vi "MISC Get Path Information.vi"(11 "Error In (no error)":errorcluster) -> (3 "Top Level VI Name":string, 4 "Root Drive":path, 6 "Application Directory":path, 8 "Support Directory":path, 10 "Top Level VI Path":path, 14 "Development Environment":bool, 15 "Error Out":errorcluster)   [LabVIEW 2017]
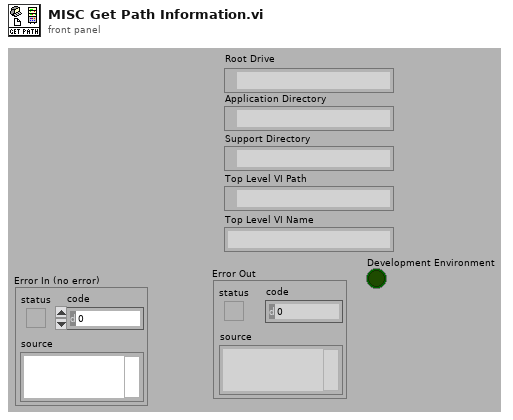
[diagram p1: front panel]
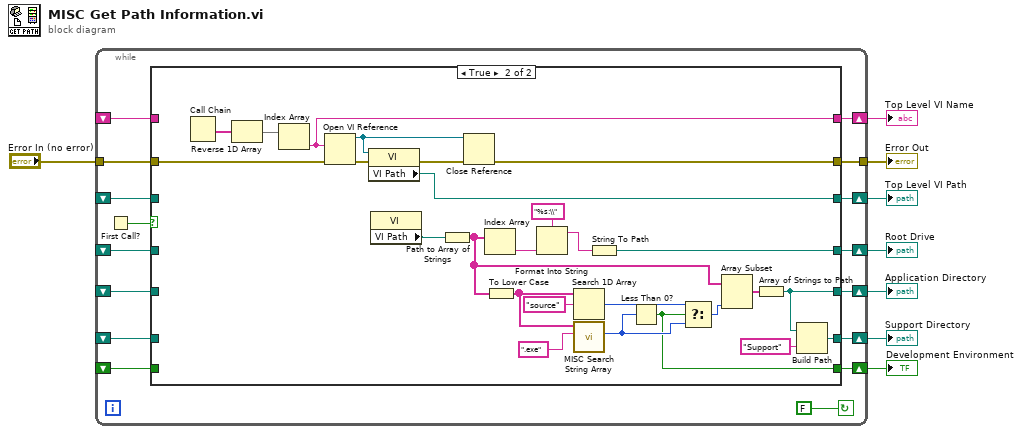
[diagram p0: block diagram]
diagram:
  n1 = while {
    tunnel: "Error In (no error)" -> [w24]
    tunnel: [w23] -> w7
    shift-right: [w17] -> w3
    shift-left: _ -> [w12]
    shift-right: [w18] -> w4
    shift-left: _ -> [w13]
    shift-right: [w19] -> w5
    shift-left: _ -> [w14]
    shift-right: [w20] -> w6
    shift-left: _ -> [w15]
    shift-right: [w21] -> w2
    shift-left: _ -> [w16]
    shift-right: [w10] -> w1
    shift-left: _ -> [w9]
    stop <- FALSE continue-if-true
    n2 = First Call?() -> (First Call?: T/F=w22:bool)
    n3 = case shown="True" w22 {
      tunnel: [w28 w57] -> w19
      tunnel: [w31 w54] -> w21
      tunnel: w24 -> [w29 w50]
      tunnel: [w29 w49] -> w23
      tunnel: [w27 w47] -> w18
      tunnel: [w26 w45] -> w17
      tunnel: [w30 w32] -> w20
      tunnel: w16 -> [w31 _]
      tunnel: w15 -> [w30 _]
      tunnel: w14 -> [w28 _]
      tunnel: w13 -> [w27 _]
      tunnel: w12 -> [w26 _]
      tunnel: [w25 w34] -> w10
      tunnel: w9 -> [w25 _]
      frame False {
      }
      frame True {
        n4 = Call Chain() -> (call chain=w56:string[])
        n5 = Reverse 1D Array(array=w56) -> (reversed array=w55:string[])
        n6 = Index Array(array=w55) -> (element=w54:string)  [unwired: 1 in]
        n7 = Open VI Reference(vi path=w54, error in (no error)=w50) -> (vi reference=w51:refnum<vi>, error out=w53:errorcluster)  [unwired: 4 out]
        n8 = property class="VI"(reference=w51, error in=w53) -> (error out=w52:errorcluster, "VI Path"=w32:path)  [unwired: 1 out]
        n9 = property class="VI"() -> ("VI Path"=w33:path)  [unwired: 2 in, 2 out]
        n10 = Path to Array of Strings(0:w33) -> (2:w44:string[])  [unwired: 1 out]
        n11 = Close Reference(reference=w51, error in (no error)=w52) -> (error out=w49:errorcluster)
        n12 = Index Array(array=w44) -> (element=w36:string)  [unwired: 1 in]
        n13 = To Lower Case(string=w44) -> (all lower case string=w42:string[])
        n14 = Format Into String(format string="%s:\\", w36) -> (resulting string=w35:string)  [unwired: 2 in, 1 out]
        n15 = Search 1D Array(1D array=w42, element="source") -> (index of element=w39:i32)  [unwired: 1 out]
        n16 = call "MISC Search String Array.vi"("String"=".exe" ("element"), "String Array"=w42) -> ("First Index"=w38:i32)  [unwired: 1 in, 8 out]
        n17 = String To Path(string=w35) -> (path=w57:path)
        n18 = Less Than 0?(x=w38) -> (x < 0?=w34:bool)
        n19 = Select(t=w39, s=w34, f=w38) -> (s? t:f=w40:i32)
        n20 = Array Subset(array=w44, length=w40) -> (w48:string[])  [unwired: 1 in]
        n21 = Array of Strings to Path(0:w48) -> (2:w47:path)  [unwired: 1 out]
        n22 = Build Path(base path=w47, name or relative path="Support") -> (appended path=w45:path)
      }
    }
  }
  "Root Drive" <- w5
  "Error Out" <- w7
  "Top Level VI Name" <- w2
  "Top Level VI Path" <- w6
  "Application Directory" <- w4
  "Support Directory" <- w3
  "Development Environment" <- w1
